vi "Water_Level_Sensor_Calibration.vi"(11 "read_in":dbl format="%0.2f") -> (3 "water level":dbl)   [LabVIEW 2022 SP3]
panel:
  out "x-y":dbl
  in  "x":dbl
  in  "y":dbl
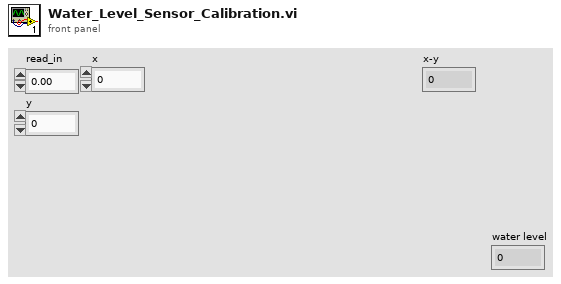
[diagram p1: front panel]
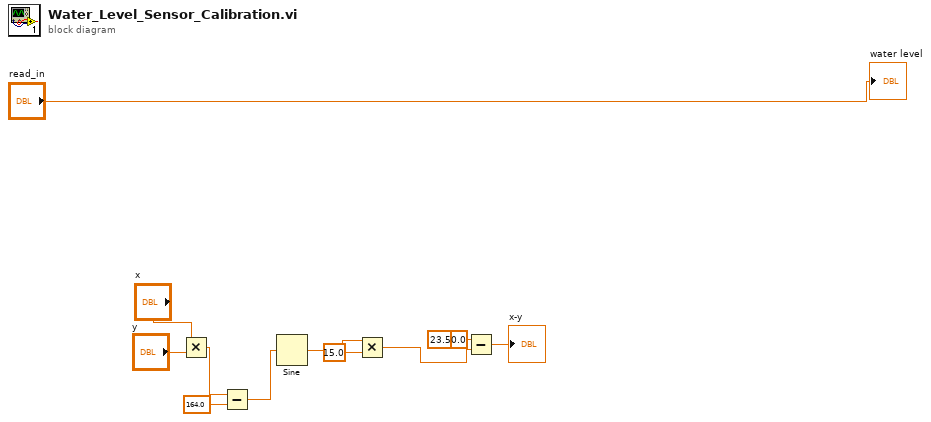
[diagram p0: block diagram]
diagram:
  (unwired) 0.0 ("x")
  n1 = Multiply(x="x", y="y") -> (x*y=w10:dbl)
  n2 = Subtract(x=w10, y=164.0) -> (x-y=w8:dbl)
  n3 = Sine(x=w8) -> (sin(x)=w7:dbl)
  n4 = Multiply(x=w7, y=15.0) -> (x*y=w5:dbl)
  n5 = Subtract(x=23.5, y=w5) -> (x-y=→"x-y":dbl)
  "water level" <- "read_in"
